vi "UDP Receiver.vi"() -> ()   [LabVIEW 2011]
panel:
  out "Data Received":string
  in  "stop":bool
  in  "Local":u16=61557
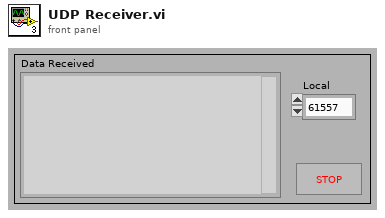
[diagram p1: front panel]
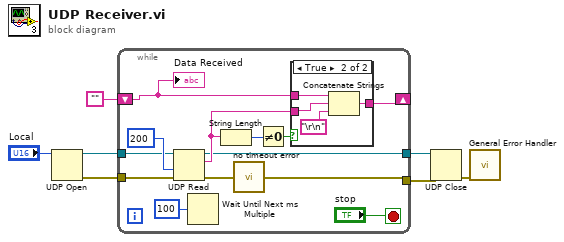
[diagram p0: block diagram]
diagram:
  n1 = UDP Open(11:"Local") -> (port=w6:refnum<k16>, 0:w5:errorcluster)  [unwired: 4 in, 1 out]
  n2 = while {
    tunnel: w6 -> [w19]
    tunnel: w5 -> [w18]
    shift-right: [w14] -> _
    shift-left: "" -> [w13]
    tunnel: [w10] -> w1
    tunnel: [w9] -> w2
    stop <- "stop" stop-if-true
    n3 = UDP Read(connection ID=w19, timeout ms (25000)=200, 8:w18) -> (data out=w12:string, error out=w11:errorcluster, 3:w9:refnum<k16>)  [unwired: 1 in, 2 out]
    n4 = Wait Until Next ms Multiple(millisecond multiple=u32 100) -> ()  [unwired: 1 out]
    n5 = String Length(string=w12) -> (length=w16:i32)
    n6 = call "no timeout error.vi"("error in (no error)"=w11) -> ("error out"=w10:errorcluster)
    n7 = Not Equal To 0?(x=w16) -> (x != 0?=w15:bool)
    n8 = case shown="True" w15 {
      tunnel: w13 -> [w21 w25]
      tunnel: w12 -> [_ w23]
      tunnel: [w21 w24] -> w14
      frame False {
      }
      frame True {
        n9 = Concatenate Strings(w25, w23, "\r\n" ("Substring")) -> (w24:string)
      }
    }
    "Data Received" <- w13
  }
  n10 = UDP Close(connection ID=w2, 8:w1) -> (error out=w3:errorcluster)  [unwired: 1 out]
  n11 = call <vilib>:"General Error Handler.vi"("error in (no error)"=w3) -> ()  [unwired: 10 in, 5 out]
